vi "USB6343_initialize_v1.2.vi"(10 "Y initial position":dbl format="%#_15g", 11 "X initial position":dbl format="%#_15g") -> (0 "error out":errorcluster caption="错误输出", 2 "interface":T2, 3 "tasks":T3)   [LabVIEW 2013]
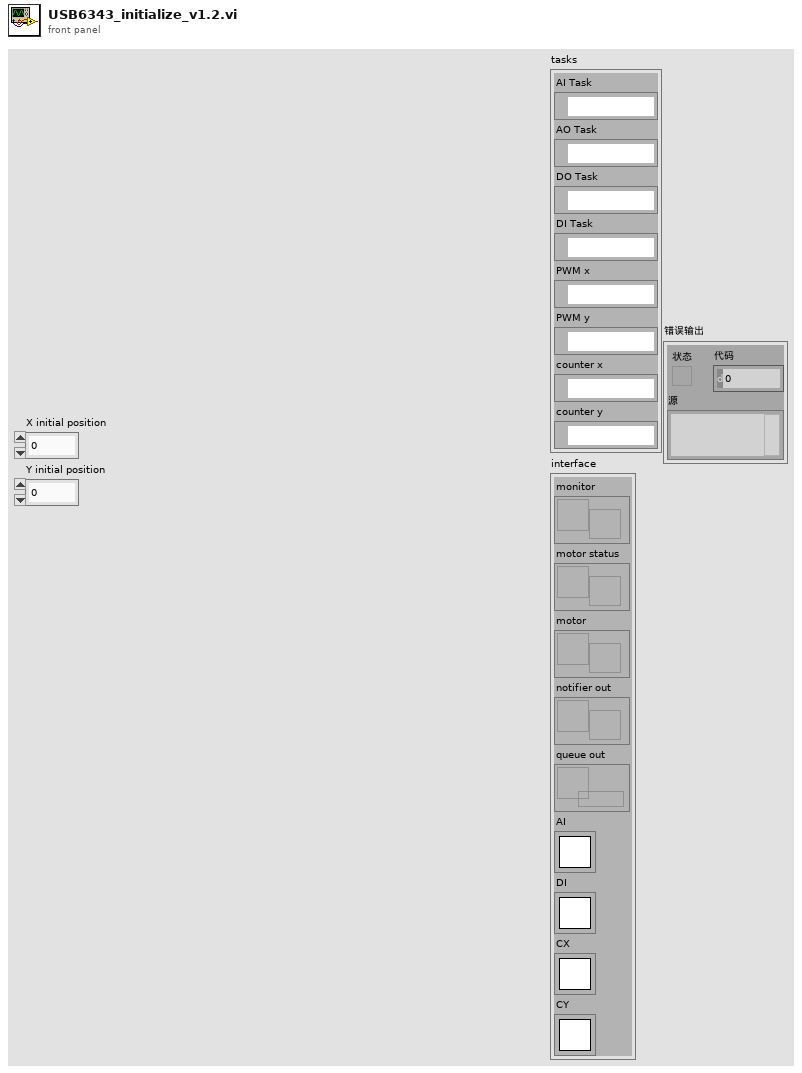
[diagram p1: front panel]
types:
  T1 = typedef "Semaphore RefNum" = refnum<k1>
  T2 = cluster{"monitor":refnum<user-event>, "motor status":refnum<user-event>, "motor":refnum<user-event>, "notifier out":refnum<notifier>, "queue out":refnum<queue>, "AI":T1, "DI":T1, "CX":T1, "CY":T1}
  T3 = cluster{"AI Task":refnum<k21>, "AO Task":refnum<k21>, "DO Task":refnum<k21>, "DI Task":refnum<k21>, "PWM x":refnum<k21>, "PWM y":refnum<k21>, "counter x":refnum<k21>, "counter y":refnum<k21>}
  T4 = cluster{"cmd":string, "channel":i32, "value":dbl, "on/off":bool, "return value":refnum<vi>}
  T5 = cluster{"monitor":refnum<user-event>, "motor status":refnum<user-event>, "motor":refnum<user-event>, "notifier out":refnum<notifier>, "queue out":refnum<queue>, "semaphore":T1, "semaphore":T1, "semaphore":T1, "semaphore":T1}
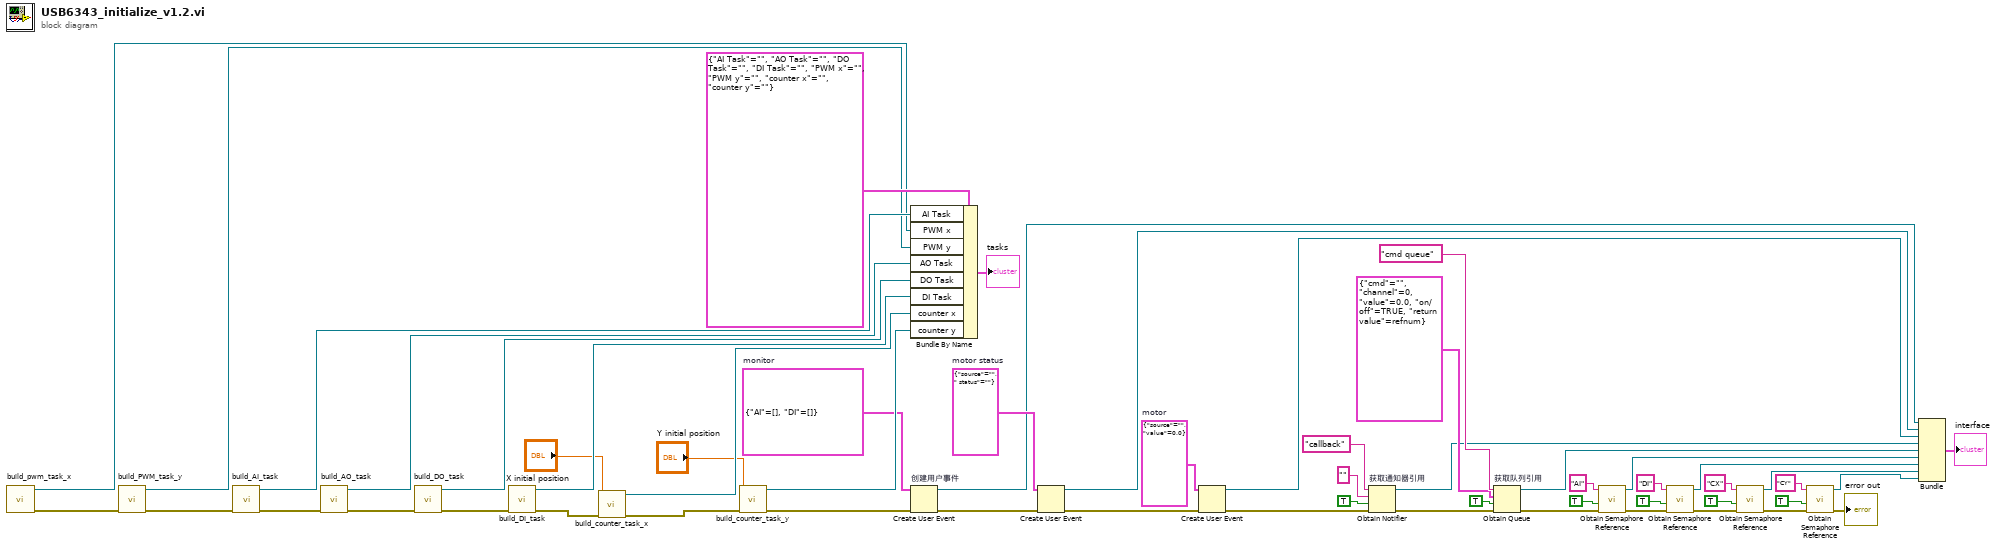
[diagram p0: block diagram]
diagram:
  w29 = cluster{"source":string, " status":string} {"source"="", " status"=""}  # motor status
  w33 = cluster{"source":string, "value":dbl} {"source"="", "value"=0.0}  # motor
  w35 = cluster{"AI":dbl[], "DI":bool[]} {"AI"=[], "DI"=[]}  # monitor
  n1 = call "build_pwm_task_x.vi"() -> ("error out"=w48:errorcluster, "task out"=w46:refnum<k21>)  [unwired: 10 in]
  n2 = call "build_PWM_task_y.vi"("error in"=w48) -> ("error out"=w47:errorcluster, "task out"=w45:refnum<k21>)  [unwired: 9 in]
  n3 = call "build_AI_task.vi"("error in"=w47) -> ("error out"=w53:errorcluster, "task out"=w55:refnum<k21>)  [unwired: 9 in]
  n4 = call "build_AO_task.vi"("error in"=w53) -> ("error out"=w51:errorcluster, "task out"=w54:refnum<k21>)  [unwired: 9 in]
  n5 = call "build_DO_task.vi"("error in"=w51) -> ("error out"=w50:errorcluster, "task out"=w49:refnum<k21>)  [unwired: 9 in]
  n6 = call "build_DI_task.vi"("error in"=w50) -> ("error out"=w44:errorcluster, "task out"=w52:refnum<k21>)  [unwired: 9 in]
  n7 = call "build_counter_task_x.vi"("error in"=w44, "initial position"="X initial position") -> ("error out"=w43:errorcluster, "task out"=w42:refnum<k21>)  [unwired: 8 in]
  n8 = call "build_counter_task_y.vi"("error in"=w43, "initial position"="Y initial position") -> ("error out"=w32:errorcluster, "task out"=w41:refnum<k21>)  [unwired: 8 in]
  n9 = Bundle By Name(cluster=T3 {"AI Task"="", "AO Task"="", "DO Task"="", "DI Task"="", "PWM x"="", "PWM y"="", "counter x"="", "counter y"=""}, "AI Task"=w55, "PWM x"=w46, "PWM y"=w45, "AO Task"=w54, "DO Task"=w49, "DI Task"=w52, "counter x"=w42, "counter y"=w41) -> (→"tasks":T3)
  n10 = Create User Event "创建用户事件"(user event datatype=w35, error in=w32) -> (user event=w12:refnum<user-event>, error out=w28:errorcluster)
  n11 = Create User Event(user event datatype=w29, error in=w28) -> (user event=w3:refnum<user-event>, error out=w27:errorcluster)
  n12 = Create User Event(user event datatype=w33, error in=w27) -> (user event=w11:refnum<user-event>, error out=w31:errorcluster)
  n13 = Obtain Notifier "获取通知器引用"(name (unnamed)="callback" ("名称（未命名）"), notification data type="", create if not found? (T)=TRUE ("如未找到是否创建？(T)"), error in (no error)=w31) -> (notifier out=w10:refnum<notifier>, error out=w30:errorcluster)  [unwired: 1 out]
  n14 = Obtain Queue "获取队列引用"(name (unnamed)="cmd queue" ("名称（未命名）"), element data type=T4 {"cmd"="", "channel"=0, "value"=0.0, "on/off"=TRUE, "return value"=refnum}, create if not found? (T)=TRUE, error in (no error)=w30) -> (queue out=w9:refnum<queue>, error out=w18:errorcluster)  [unwired: 1 in, 1 out]
  n15 = call <vilib>:"Obtain Semaphore Reference.vi"("error in (no error)"=w18, "create if not found (T)"=TRUE, "name (unnamed)"="AI") -> ("error out"=w21:errorcluster, "semaphore"=w8:T1)  [unwired: 2 in, 1 out]
  n16 = call <vilib>:"Obtain Semaphore Reference.vi"("error in (no error)"=w21, "create if not found (T)"=TRUE, "name (unnamed)"="DI") -> ("error out"=w20:errorcluster, "semaphore"=w7:T1)  [unwired: 2 in, 1 out]
  n17 = call <vilib>:"Obtain Semaphore Reference.vi"("error in (no error)"=w20, "create if not found (T)"=TRUE, "name (unnamed)"="CX") -> ("error out"=w19:errorcluster, "semaphore"=w6:T1)  [unwired: 2 in, 1 out]
  n18 = call <vilib>:"Obtain Semaphore Reference.vi"("error in (no error)"=w19, "create if not found (T)"=TRUE, "name (unnamed)"="CY") -> ("error out"=→"error out":errorcluster, "semaphore"=w5:T1)  [unwired: 2 in, 1 out]
  n19 = Bundle("monitor"=w12, "motor status"=w3, "motor"=w11, "notifier out"=w10, "queue out"=w9, "semaphore"=w8, "semaphore"=w7, "semaphore"=w6, "semaphore"=w5) -> (→"interface":T5)  [unwired: 1 in]
